vi "Return MutationCode Folder.vi"() -> (3 "Base Path Mutation Code":path)   [LabVIEW 2017, in "lv_icon.lvlib"]
uses:
  <vilib>/LabVIEW Icon API/lv_icon/lv_icon.lvlib
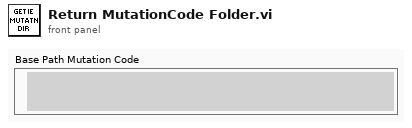
[diagram p1: front panel]
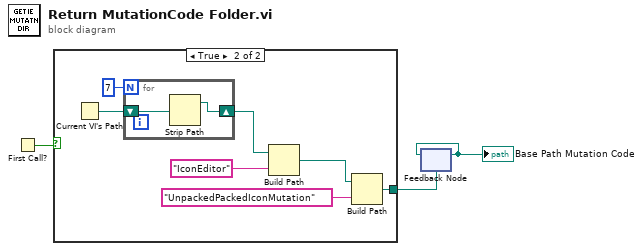
[diagram p0: block diagram]
diagram:
  n1 = First Call?() -> (First Call?: T/F=w1:bool)
  n2 = case shown="True" w1 {
    tunnel: [_ w6] -> w3
    frame False {
    }
    frame True {
      n3 = Current VI's Path() -> (path=w5:path)
      n4 = for {
        N: 7 -> [_]
        shift-right: [w11] -> w10
        shift-left: w5 -> [w12]
        n5 = Strip Path(path=w12) -> (stripped path=w11:path)  [unwired: 1 out]
      }
      n6 = Build Path(base path=w10, name or relative path="IconEditor") -> (appended path=w7:path)
      n7 = Build Path(base path=w7, name or relative path="UnpackedPackedIconMutation") -> (appended path=w6:path)
    }
  }
  n8 = feedback #1(w3) -> (w2:path)
  "Base Path Mutation Code" <- w2
  n9 = feedback-in #1(w2) -> ()
